vi "EMI_project.vi"() -> ()   [LabVIEW 2020]
uses:
  <vilib>/Instr/_visa.llb/VISA Configure Serial Port (Instr).vi
panel:
  in  "Calibrate":bool
  in  "stop":bool
  in  "VISA resource name":refnum<visa-resource-name>
  in  "?":bool
  in  "Gain02":bool
  in  "?":bool
  in  "Gain01":bool
  in  "?":bool
  in  "Fader02":bool
  in  "?":bool
  in  "Fader01":bool
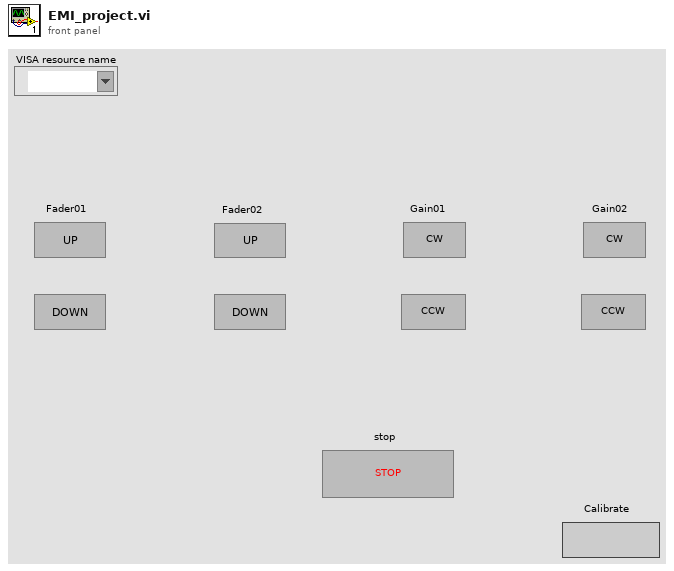
[diagram p1: front panel]
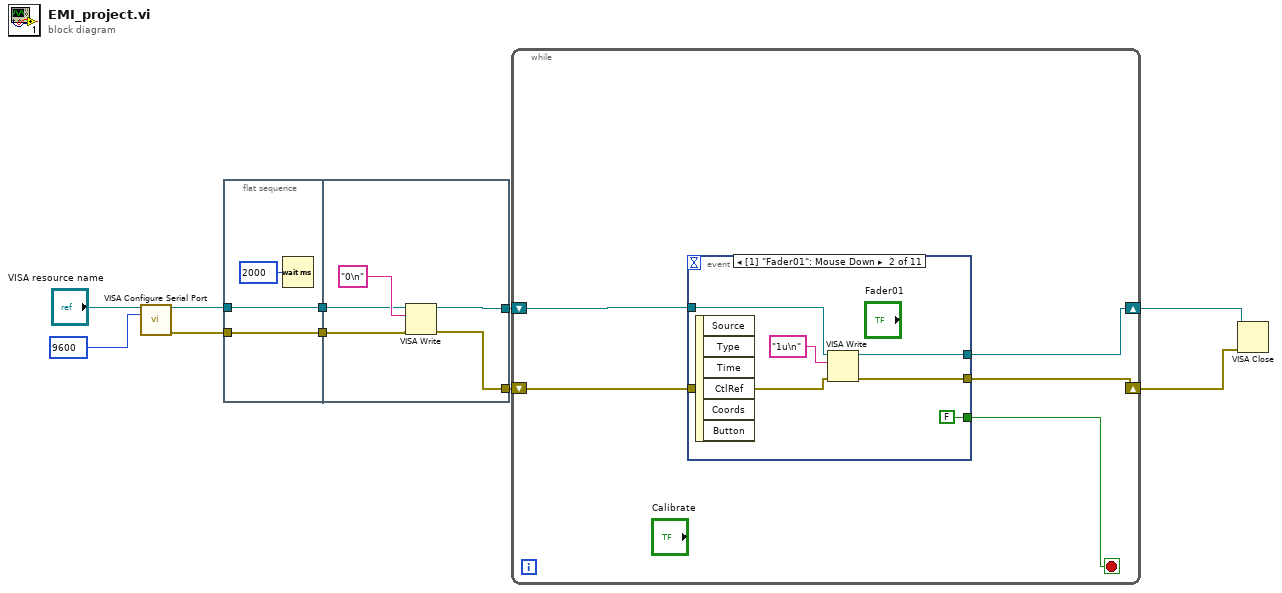
[diagram p0: block diagram]
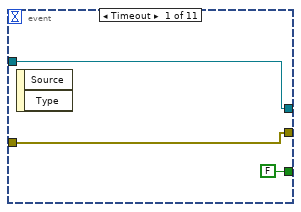
[diagram p2: hidden frame]
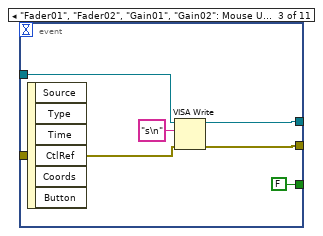
[diagram p3: hidden frame]
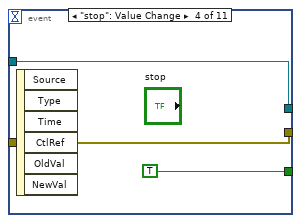
[diagram p4: hidden frame]
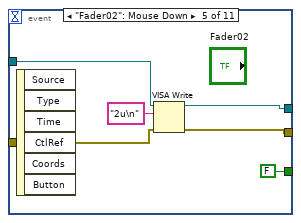
[diagram p5: hidden frame]
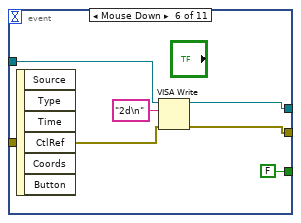
[diagram p6: hidden frame]
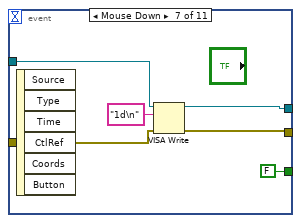
[diagram p7: hidden frame]
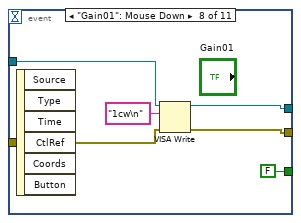
[diagram p8: hidden frame]
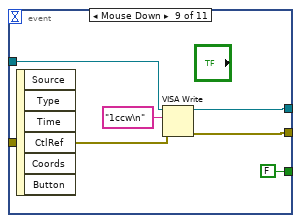
[diagram p9: hidden frame]
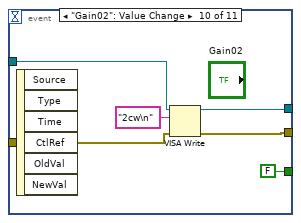
[diagram p10: hidden frame]
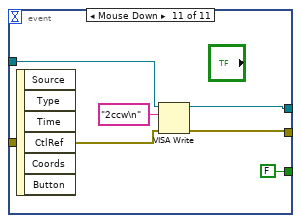
[diagram p11: hidden frame]
diagram:
  n1 = call-poly "VISA Configure Serial Port"("VISA resource name"="VISA resource name", "baud rate (9600)"=u32 9600) -> ("VISA resource name out"=w4:refnum<visa-resource-name>, "error out"=w3:errorcluster)  [unwired: 12 in]
  n2 = flat-sequence {
    tunnel: w3 -> [w12]
    tunnel: w4 -> [w13]
    tunnel: [w13] -> w2
    tunnel: [w12] -> w1
    tunnel: [w17] -> w8
    tunnel: [w16] -> w7
    tunnel: w2 -> [w15]
    tunnel: w1 -> [w14]
    frame #0 {
      n3 = Wait (ms)(milliseconds to wait=u32 2000) -> ()  [unwired: 1 out]
    }
    frame #1 {
      n4 = VISA Write(VISA resource name=w15, write buffer="0\n", error in (no error)=w14) -> (VISA resource name out=w17:refnum<visa-resource-name>, error out=w16:errorcluster)  [unwired: 1 out]
    }
  }
  n5 = while {
    shift-right: [w21] -> w6
    shift-left: w8 -> [w23]
    shift-right: [w20] -> w5
    shift-left: w7 -> [w22]
    stop <- w19 stop-if-true
    n6 = event shown="[1] \"Fader01\": Mouse Down" {
      selector: _ -> [_ _ _ _ _ _ _ _ _ _ _]
      dyn-events: _ -> [_ _ _ _ _ _ _ _ _ _ _]
      timeout: _ -> [_ _ _ _ _ _ _ _ _ _ _]
      tunnel: w23 -> [w26 w32 w36 w40 w45 w51 w59 w63 w68 w75 w81]
      tunnel: w22 -> [w25 w31 w35 w39 w44 w50 w58 w62 w69 w74 w80]
      tunnel: [w26 w29 w38 w40 w47 w53 w56 w65 w71 w77 w83] -> w21
      tunnel: [w25 w28 w37 w39 w46 w52 w57 w64 w70 w76 w82] -> w20
      tunnel: [FALSE FALSE FALSE TRUE FALSE FALSE FALSE FALSE FALSE FALSE FALSE] -> w19
      event Timeout {
        n7 = event-data() -> ()  [unwired: 1 in, 2 out]
      }
      event "Fader01": Mouse Down {
        n8 = event-data() -> ()  [unwired: 1 in, 6 out]
        n9 = VISA Write(VISA resource name=w32, write buffer="1u\n", error in (no error)=w31) -> (VISA resource name out=w29:refnum<visa-resource-name>, error out=w28:errorcluster)  [unwired: 1 out]
      }
      event "Fader01", "Fader02", "Gain01", "Gain02": Mouse Up {
        n10 = event-data() -> ()  [unwired: 1 in, 6 out]
        n11 = VISA Write(VISA resource name=w36, write buffer="s\n", error in (no error)=w35) -> (VISA resource name out=w38:refnum<visa-resource-name>, error out=w37:errorcluster)  [unwired: 1 out]
      }
      event "stop": Value Change {
        n12 = event-data() -> ()  [unwired: 1 in, 6 out]
      }
      event "Fader02": Mouse Down {
        n13 = event-data() -> ()  [unwired: 1 in, 6 out]
        n14 = VISA Write(VISA resource name=w45, write buffer="2u\n", error in (no error)=w44) -> (VISA resource name out=w47:refnum<visa-resource-name>, error out=w46:errorcluster)  [unwired: 1 out]
      }
      event Mouse Down {
        n15 = event-data() -> ()  [unwired: 1 in, 6 out]
        n16 = VISA Write(VISA resource name=w51, write buffer="2d\n", error in (no error)=w50) -> (VISA resource name out=w53:refnum<visa-resource-name>, error out=w52:errorcluster)  [unwired: 1 out]
      }
      event Mouse Down {
        n17 = event-data() -> ()  [unwired: 1 in, 6 out]
        n18 = VISA Write(VISA resource name=w59, write buffer="1d\n", error in (no error)=w58) -> (VISA resource name out=w56:refnum<visa-resource-name>, error out=w57:errorcluster)  [unwired: 1 out]
      }
      event "Gain01": Mouse Down {
        n19 = event-data() -> ()  [unwired: 1 in, 6 out]
        n20 = VISA Write(VISA resource name=w63, write buffer="1cw\n", error in (no error)=w62) -> (VISA resource name out=w65:refnum<visa-resource-name>, error out=w64:errorcluster)  [unwired: 1 out]
      }
      event Mouse Down {
        n21 = event-data() -> ()  [unwired: 1 in, 6 out]
        n22 = VISA Write(VISA resource name=w68, write buffer="1ccw\n", error in (no error)=w69) -> (VISA resource name out=w71:refnum<visa-resource-name>, error out=w70:errorcluster)  [unwired: 1 out]
      }
      event "Gain02": Value Change {
        n23 = event-data() -> ()  [unwired: 1 in, 6 out]
        n24 = VISA Write(VISA resource name=w75, write buffer="2cw\n", error in (no error)=w74) -> (VISA resource name out=w77:refnum<visa-resource-name>, error out=w76:errorcluster)  [unwired: 1 out]
      }
      event Mouse Down {
        n25 = event-data() -> ()  [unwired: 1 in, 6 out]
        n26 = VISA Write(VISA resource name=w81, write buffer="2ccw\n", error in (no error)=w80) -> (VISA resource name out=w83:refnum<visa-resource-name>, error out=w82:errorcluster)  [unwired: 1 out]
      }
    }
  }
  n27 = VISA Close(VISA resource name=w6, error in (no error)=w5) -> ()  [unwired: 1 out]
